vi "Write Spectrum Analyzer.lvclass.vi"(10 "Spectrum Analyzer.lvclass":refnum<class "Spectrum Analyzer.lvclass">, 11 "IMD in":refnum<class "IMD.lvclass">) -> (3 "IMD out":refnum<class "IMD.lvclass">)   [LabVIEW 2020, in "IMD.lvclass"]
uses:
  IMD.lvclass
  Instruments/Spectrum Analyzer/Spectrum Analyzer.lvclass
  IMD.lvclass/IMD.ctl
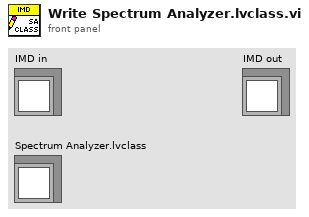
[diagram p1: front panel]
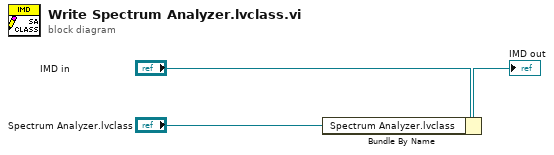
[diagram p0: block diagram]
diagram:
  n1 = Bundle By Name(cluster="IMD in", "Spectrum Analyzer.lvclass"="Spectrum Analyzer.lvclass") -> (→"IMD out":refnum<class "IMD.lvclass">)
